vi "Teleop.vi"(10 "Match Info":T1={"Autonomous Elapsed Seconds"=0.0, "TeleOp Elapsed Seconds"=0.0, "Disabled Elapsed Seconds"=0.0, "Visited Autonomous"=FALSE, "Visited TeleOp"=FALSE, "Visited Disabled"=FALSE, "Autonomous Settings"={"Autonomous Style"=enum."Independent", "VI Refnum"=refnum}}, 11 "Call Context":T2) -> ()   [LabVIEW 2012]
doc: "This VI is called for each TeleOp packet received from the DS where the robot is not disabled. It is often used to read from the joysticks and update I/O or to update setpoints for timed control loops. It should complete and return within 20 milliseconds or it may miss DS packets."
uses:
  <vilib>/Rock Robotics/WPI/DriverStation/WPI_DriverStationDerivedRobotMode.ctl
  <vilib>/Rock Robotics/WPI/DriverStation/WPI_DriverStationMatch Info.ctl
  Robot Global Data.vi
  <vilib>/Rock Robotics/WPI/Joystick/WPI_JoystickGetSetRefNum.vi
  <vilib>/Rock Robotics/WPI/RobotDrive/WPI_RobotDriveGetSetRefNum.vi
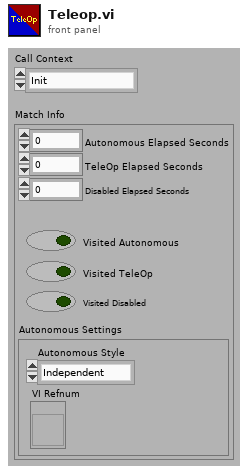
[diagram p1: front panel]
types:
  T1 = typedef "WPI_DriverStationMatch Info.ctl" = cluster{"Autonomous Elapsed Seconds":dbl, "TeleOp Elapsed Seconds":dbl, "Disabled Elapsed Seconds":dbl, "Visited Autonomous":bool, "Visited TeleOp":bool, "Visited Disabled":bool, "Autonomous Settings":cluster{"Autonomous Style":enum16{"Iterative", "Independent"}, "VI Refnum":refnum<vi>}}
  T2 = typedef "WPI_DriverStationDerivedRobotMode.ctl" = enum16{"Init", "Execute", "Stop"}
  T3 = typedef "WPI_JoystickDevRef.ctl" = cluster{"Device":T4}
  T4 = typedef "WPI_JoystickDeviceEnum.ctl" = enum16{"USB 1", "USB 2", "USB 3", "USB 4", "Kinect 1", "Kinect 2"}
  T5 = typedef "WPI_JoystickButtonState.ctl" = cluster{"Button 1":bool, "Button 2":bool, "Button 3":bool, "Button 4":bool, "Button 5":bool, "Button 6":bool, "Button 7":bool, "Button 8":bool, "Button 9":bool, "Button 10":bool, "Button 11":bool, "Button 12":bool}
  T6 = cluster{"axis 1 (x)":dbl, "axis 2 (y)":dbl, "axis 3 (throttle)":dbl, "axis 4":dbl, "axis 5":dbl, "axis 6":dbl}
  T7 = typedef "WPI_RobotDriveDevRef.ctl" = cluster{"DevStatus":errorcluster, "Motors[]":T8[], "Square Inputs":bool, "Max Output":dbl, "Isochronous":bool}
  T8 = typedef "WPI_MotorControlDeviceRef.ctl" = cluster{"DeviceStatus":errorcluster, "Type":enum16{"PWM", "CAN"}, "PWM":cluster{"Digital Module":T9, "PWM Channel":T10, "DeadBand":T11}, "CAN":cluster{"Device Number":u8, "Control Mode":T12, "Semaphore":T13, "Max Vout":dbl}, "Invert":bool, "TransformRef":T14, "InvTransformRef":T14}
  T9 = typedef "FPGA_TypedefDigitalModule.ctl" = enum16{"Digital Module 1", "Digital Module 2"}
  T10 = typedef "FPGA_DIOPWMChannel.ctl" = enum8{"PWM 1", "PWM 2", "PWM 3", "PWM 4", "PWM 5", "PWM 6", "PWM 7", "PWM 8", "PWM 9", "PWM 10", "Invalid"}
  T11 = typedef "WPI_PWMDeadband.ctl" = cluster{"Name":string, "maxPositivePwm":i32, "minPositivePwm":i32, "centerPwm":i32, "maxNegativePwm":i32, "minNegativePwm":i32, "angularRange":u16}
  T12 = typedef "WPI_CANJaguar_ControlMode.ctl" = enum8{"Percent VBus", "Current", "Speed", "Position", "Voltage"}
  T13 = typedef "Semaphore RefNum" = refnum<k1>
  T14 = typedef "WPI_PWMTransform_ConPane.ctl" = refnum<vi>
  T15 = cluster{"Shoot":bool, "Enable_Targeting":bool, "Shooter":dbl, "LeadScrew":dbl, "Feed":bool, "Pickup":bool, "LiftHooks":bool, "Vision On":bool, "Vision Off":bool, "DownHooks":bool}
  T16 = cluster{"PizzaLow":dbl, "PizzaMid":dbl, "PizzaTop":dbl}
  T17 = typedef "WPI_DigitalInputDevRef.ctl" = cluster{"DevStatus":errorcluster, "DIO Channel":T18, "Digital Module":T9}
  T18 = typedef "FPGA_DIOChannel.ctl" = enum8{"DIO 1", "DIO 2", "DIO 3", "DIO 4", "DIO 5", "DIO 6", "DIO 7", "DIO 8", "DIO 9", "DIO 10", "DIO 11", "DIO 12", "DIO 13", "DIO 14", "Invalid"}
  T19 = cluster{"Frisbee_Catch":bool, "Shooter_Ready":bool, "LeadScrewEnd":bool}
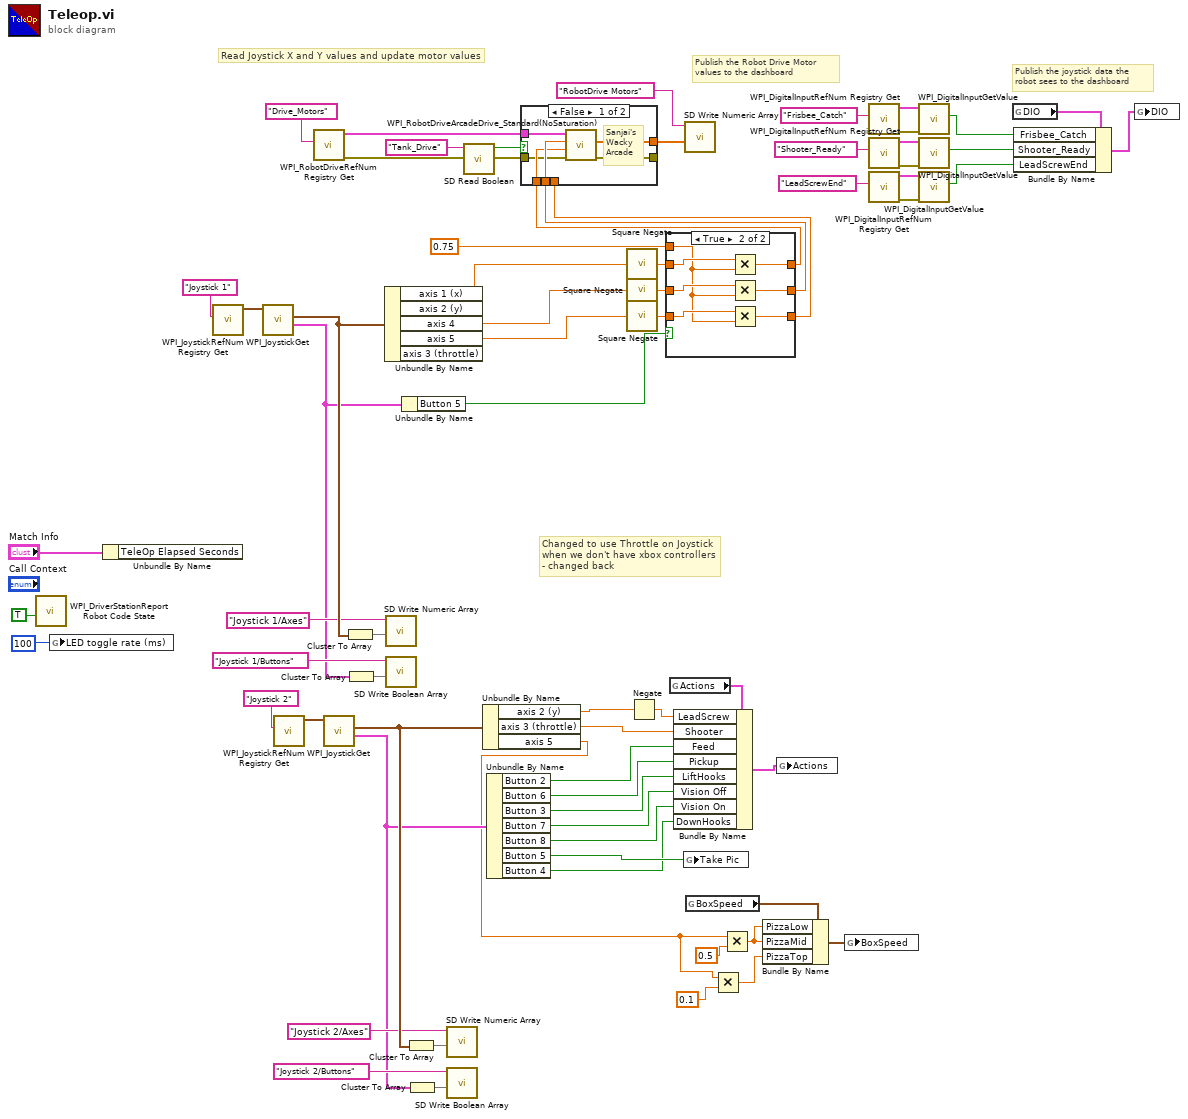
[diagram p0: block diagram]
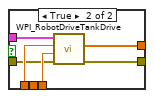
[diagram p3: hidden frame]
diagram:
  # "Changed to use Throttle on Joystick\nwhen we don't have xbox controllers\n- changed back"
  # "Publish the Robot Drive Motor\nvalues to the dashboard"
  # "Publish the joystick data the\nrobot sees to the dashboard"
  # "Read Joystick X and Y values and update motor values"
  n1 = call <vilib>:"WPI_DriverStationReport Robot Code State.vi"("TeleOp"=TRUE ("Autonomous")) -> ()  [unwired: 10 in, 1 out]
  n2 = global write "Robot Global Data.vi" "LED toggle rate (ms)"(u32 100 ("LED ms toggle rate")) -> ()
  n3 = Unbundle By Name("Match Info") -> ()  [unwired: 1 out]
  n4 = call <vilib>:"WPI_JoystickRefNum Registry Get.vi"("refnum name"="Joystick 1") -> ("JoystickDevRef"=w65:T3)  [unwired: 1 in, 9 out]
  n5 = call <vilib>:"WPI_JoystickGet.vi"("JoystickDevRef"=w65) -> ("Buttons"=w55:T5, "Axes"=w62:T6)  [unwired: 1 in, 4 out]
  n6 = call <vilib>:"WPI_JoystickRefNum Registry Get.vi"("refnum name"="Joystick 2") -> ("JoystickDevRef"=w44:T3)  [unwired: 1 in, 9 out]
  n7 = call <vilib>:"WPI_RobotDriveRefNum Registry Get.vi"("refnum name"="Drive_Motors") -> ("error out"=w2:errorcluster, "RobotDriveDevRef"=w67:T7)  [unwired: 1 in, 8 out]
  n8 = call <vilib>:"WPI_JoystickGet.vi"("JoystickDevRef"=w44) -> ("Buttons"=w38:T5, "Axes"=w41:T6)  [unwired: 1 in, 4 out]
  n9 = Cluster To Array(cluster=w62) -> (array=w61:dbl[])
  n10 = Cluster To Array(cluster=w55) -> (array=w64:bool[])
  n11 = Unbundle By Name(w62) -> ("axis 2 (y)"=w18:dbl, "axis 4"=w10:dbl, "axis 5"=w13:dbl)  [unwired: 2 out]
  n12 = call <vilib>:"SD Write Numeric Array.vi"("Numeric Array"=w61, "Name"="Joystick 1/Axes") -> ()  [unwired: 8 in, 2 out]
  n13 = call <vilib>:"SD Write Boolean Array.vi"("Boolean Array"=w64, "Name"="Joystick 1/Buttons") -> ()  [unwired: 8 in, 2 out]
  n14 = Unbundle By Name(w55) -> ("Button 5"=w35:bool)
  n15 = Cluster To Array(cluster=w41) -> (array=w40:dbl[])
  n16 = Cluster To Array(cluster=w38) -> (array=w43:bool[])
  n17 = call <vilib>:"SD Write Numeric Array.vi"("Numeric Array"=w40, "Name"="Joystick 2/Axes") -> ()  [unwired: 8 in, 2 out]
  n18 = call <vilib>:"SD Write Boolean Array.vi"("Boolean Array"=w43, "Name"="Joystick 2/Buttons") -> ()  [unwired: 8 in, 2 out]
  n19 = call <vilib>:"SD Read Boolean.vi"("Name"="Tank_Drive") -> ("Boolean"=w57:bool)  [unwired: 8 in, 2 out]
  n20 = Unbundle By Name(w41) -> ("axis 2 (y)"=w27:dbl, "axis 3 (throttle)"=w28:dbl, "axis 5"=w1:dbl)
  n21 = Unbundle By Name(w38) -> ("Button 2"=w12:bool, "Button 6"=w11:bool, "Button 3"=w9:bool, "Button 7"=w8:bool, "Button 8"=w7:bool, "Button 5"=w4:bool, "Button 4"=w3:bool)
  n22 = call "Square Negate.vi"("x"=w18) -> ("x脖"=w19:dbl)
  n23 = call "Square Negate.vi"("x"=w10) -> ("x脖"=w17:dbl)
  n24 = call "Square Negate.vi"("x"=w13) -> ("x脖"=w20:dbl)
  n25 = Negate(x=w27) -> (-x=w26:dbl)
  n26 = case shown="True" w35 {
    tunnel: w19 -> [w71 w80]
    tunnel: w20 -> [w72 w79]
    tunnel: w17 -> [w73 w78]
    tunnel: [w73 w75] -> w15
    tunnel: [w71 w77] -> w16
    tunnel: [w72 w76] -> w14
    tunnel: 0.75 -> [_ w74]
    frame False {
    }
    frame True {
      n27 = Multiply(x=w80, y=w74) -> (x*y=w77:dbl)
      n28 = Multiply(x=w78, y=w74) -> (x*y=w75:dbl)
      n29 = Multiply(x=w79, y=w74) -> (x*y=w76:dbl)
    }
  }
  n30 = case shown="False" w57 {
    tunnel: w67 -> [w86 w91]
    tunnel: [w85 w92] -> w58
    tunnel: w14 -> [_ w90]
    tunnel: w15 -> [w84 _]
    tunnel: w16 -> [w83 w89]
    tunnel: w2 -> [w82 w88]
    tunnel: [w81 w87] -> _
    frame False {
      # "Sanjai's\nWacky\nArcade"
      n31 = call <vilib>:"WPI_RobotDriveArcadeDrive_Standard(NoSaturation).vi"("error in (no error)"=w82, "Y axis value"=w83, "X axis value"=w84, "RobotDriveDevRef"=w86) -> ("error out"=w81:errorcluster, "Motor Values"=w85:dbl[])  [unwired: 6 out]
    }
    frame True {
      n32 = call <vilib>:"WPI_RobotDriveTankDrive.vi"("error in (no error)"=w88, "Right axis value"=w90, "Left axis value"=w89, "RobotDriveDevRef"=w91) -> ("error out"=w87:errorcluster, "Motor Values"=w92:dbl[])  [unwired: 5 in, 1 out]
    }
  }
  n33 = global read "Robot Global Data.vi" "Actions"() -> (w30:T15)
  n34 = Bundle By Name(cluster=w30, "LeadScrew"=w26, "Shooter"=w28, "Feed"=w12, "Pickup"=w11, "LiftHooks"=w9, "Vision Off"=w8, "Vision On"=w7, "DownHooks"=w3) -> (w29:T15)
  n35 = global write "Robot Global Data.vi" "Take Pic"(w4) -> ()
  n36 = call <vilib>:"SD Write Numeric Array.vi"("Numeric Array"=w58, "Name"="RobotDrive Motors") -> ()  [unwired: 8 in, 2 out]
  n37 = global read "Robot Global Data.vi" "BoxSpeed"() -> (w25:T16)
  n38 = Multiply(x=w1, y=0.1) -> (x*y=w6:dbl)
  n39 = Multiply(x=w1, y=0.5) -> (x*y=w23:dbl)
  n40 = Bundle By Name(cluster=w25, "PizzaLow"=w23, "PizzaMid"=w23, "PizzaTop"=w6) -> (w24:T16)
  n41 = global write "Robot Global Data.vi" "Actions"(w29) -> ()
  n42 = global write "Robot Global Data.vi" "BoxSpeed"(w24) -> ()
  n43 = call <vilib>:"WPI_DigitalInputRefNum Registry Get.vi"("refnum name"="Frisbee_Catch") -> ("error out"=w46:errorcluster, "DigitalInputDevRef"=w47:T17)  [unwired: 9 in]
  n44 = call <vilib>:"WPI_DigitalInputRefNum Registry Get.vi"("refnum name"="Shooter_Ready") -> ("error out"=w49:errorcluster, "DigitalInputDevRef"=w48:T17)  [unwired: 9 in]
  n45 = call <vilib>:"WPI_DigitalInputRefNum Registry Get.vi"("refnum name"="LeadScrewEnd") -> ("error out"=w33:errorcluster, "DigitalInputDevRef"=w32:T17)  [unwired: 9 in]
  n46 = call <vilib>:"WPI_DigitalInputGetValue.vi"("error in (no error)"=w46, "DigitalInputDevRef"=w47) -> ("Value"=w22:bool)  [unwired: 7 in, 2 out]
  n47 = call <vilib>:"WPI_DigitalInputGetValue.vi"("error in (no error)"=w49, "DigitalInputDevRef"=w48) -> ("Value"=w45:bool)  [unwired: 7 in, 2 out]
  n48 = call <vilib>:"WPI_DigitalInputGetValue.vi"("error in (no error)"=w33, "DigitalInputDevRef"=w32) -> ("Value"=w31:bool)  [unwired: 7 in, 2 out]
  n49 = global read "Robot Global Data.vi" "DIO"() -> (w53:T19)
  n50 = Bundle By Name(cluster=w53, "Frisbee_Catch"=w22, "Shooter_Ready"=w45, "LeadScrewEnd"=w31) -> (w52:T19)
  n51 = global write "Robot Global Data.vi" "DIO"(w52) -> ()
